vi "Read Account File.vi"(8 "error in (no error)":errorcluster, 11 "ATM Data":T1) -> (0 "error out":errorcluster, 3 "ATM Data Out":T1)   [LabVIEW 2020, in "ATM Machine.lvlib"]
uses:
  ATM Machine.lvlib
  Cluster - ATM Machine Data.ctl
  Users/khemr/OneDrive/Desktop/Labview Training/CLD/New ATM_KR/ATM Machine/Cluster - Message Cluster.ctl
  Enum - ATM States.ctl
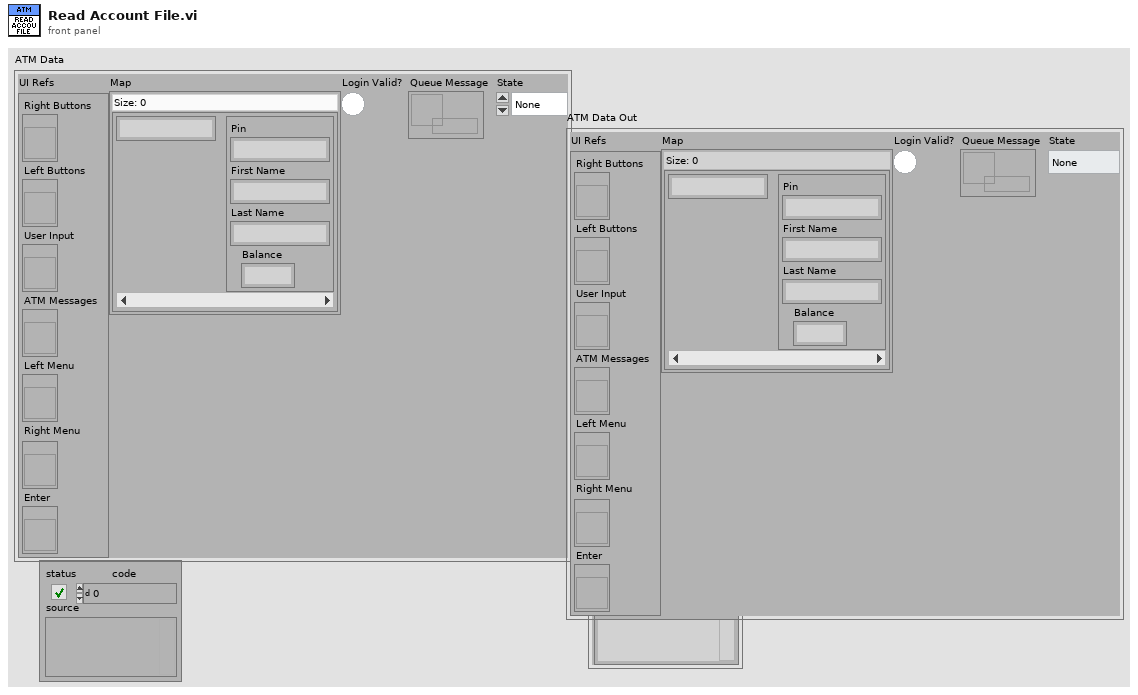
[diagram p1: front panel]
types:
  T1 = typedef "ATM Machine.lvlib/Cluster - ATM Machine Data.ctl" = cluster{"UI Refs":cluster{"Right Buttons":refnum<vi>, "Left Buttons":refnum<vi>, "User Input":refnum<vi>, "ATM Messages":refnum<vi>, "Left Menu":refnum<vi>, "Right Menu":refnum<vi>, "Enter":refnum<vi>}, "Map":map{string, cluster{"Pin":string, "First Name":string, "Last Name":string, "Balance":dbl}}, "Login Valid?":bool, "Queue Message":refnum<queue>, "State":T2}
  T2 = typedef "ATM Machine.lvlib/Enum - ATM States.ctl" = enum16{"None", "Deposit", "Withdraw", "Card Inserted", "Balance Inquiry", "Return Card and Terminate", "Fast Cash"}
  T3 = map{string, cluster{"Pin":string, "First Name":string, "Last Name":string, "Balance":dbl}}
  T4 = cluster{"Pin":string, "First Name":string, "Last Name":string, "Balance":dbl}
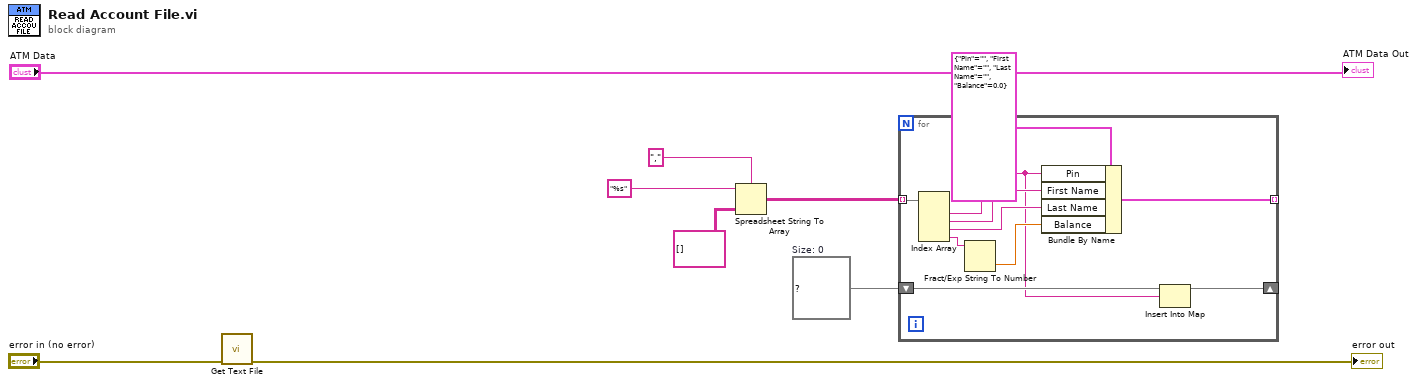
[diagram p0: block diagram]
diagram:
  w3 = T3 {}  # Size: 0
  n1 = call "Get Text File.vi"("error in (no error)"="error in (no error)") -> ("error out"=→"error out":errorcluster)  [unwired: 9 in, 1 out]
  n2 = Spreadsheet String To Array(delimiter (Tab)=",", format string="%s", array type (2D Dbl)=string[][] []) -> (array=w4:string[][])  [unwired: 1 in]
  n3 = for {
    tunnel: w4 -> [w17] mode=indexing
    shift-right: [w11] -> _
    shift-left: w3 -> [w12]
    tunnel: [w9] -> _ mode=indexing
    n4 = Index Array(array=w17) -> (element #1=w10:string, element #2=w16:string, element #3=w15:string, element #4=w14:string)  [unwired: 4 in]
    n5 = Fract/Exp String To Number(string=w14) -> (number=w13:dbl)  [unwired: 3 in, 1 out]
    n6 = Bundle By Name(cluster=T4 {"Pin"="", "First Name"="", "Last Name"="", "Balance"=0.0}, "Pin"=w10, "First Name"=w16, "Last Name"=w15, "Balance"=w13) -> (w9:T4)
    n7 = Insert Into Map(map in=w12, key=w10) -> (map out=w11:T3)  [unwired: 1 in, 2 out]
  }
  "ATM Data Out" <- "ATM Data"
